vi "Get Shutter Min Times.vi"(10 "minopeningtime":i32, 11 "minclosingtime":i32) -> (1 "function return":u32, 2 "minopeningtime out":i32, 3 "minclosingtime out":i32)   [LabVIEW 2018, in "Copy of Andor SDK.lvlib"]
doc: "EXPNETTYPE unsigned int WINAPI GetShutterMinTimes(int * minclosingtime, int * minopeningtime);"
uses:
  Copy of Andor SDK.lvlib
  <userlib>/Andor SDK/ATMCD32D.dll
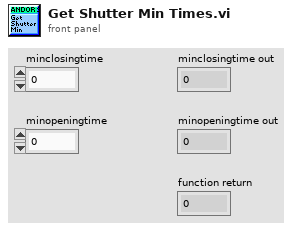
[diagram p1: front panel]
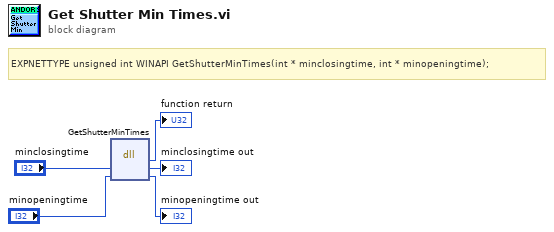
[diagram p0: block diagram]
diagram:
  # "EXPNETTYPE unsigned int WINAPI GetShutterMinTimes(int * minclosingtime, int * minopeningtime);"
  n1 = dll-call lib="C:/Program Files (x86)/National Instruments/LabVIEW 2018/user.lib/Andor SDK/ATMCD32D.*" fn="GetShutterMinTimes"("minclosingtime"="minclosingtime", "minopeningtime"="minopeningtime") -> (→"function return":u32, "minclosingtime"=→"minclosingtime out":i32, "minopeningtime"=→"minopeningtime out":i32)  [unwired: 3 in, 2 out]
